vi "Not Equivalent.vi"(8 "Other JSON":string="{}", 10 "JSON":string="{}") -> (2 "Not Equivalent":bool caption="Not Equivalent (or invalid)")   [LabVIEW 2019, in "JSONtext.lvlib"]
doc: "Returns True if two JSON Values are \"Not Equivalent\".\n\nEqual means they are the same JSON infomation. Not considered differences are:\n -- different order of JSON Object items\n -- presence of any formating whitespace (outside of a JSON String)\n -- different formating of numbers (123.00 verus 123 or 1.23E2)\n\nNote: If using the LabVIEW extension that uses NaN numbers, these are considered Equivalent, ignoring the ususal convention of NaN not equal to NaN.\n\nInvalid JSON will always return \"Not Equivalent\" even if both inputs are identical.\n\nThis function looks only at the leading JSON Value in the input strings, ignoring any following characters."
uses:
  JSONtext.lvlib
  support/Get Number Text.vi
  String Subset.vi
  Parsing/Advance past Number.vi
  Parsing/Parsing Error in converting to LabVIEW type.vi
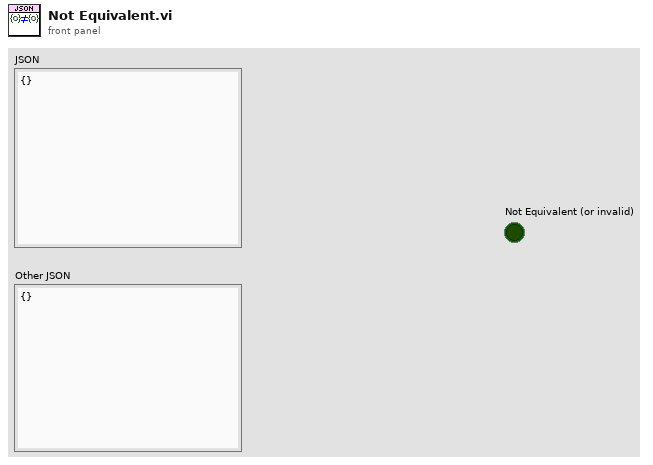
[diagram p1: front panel]
types:
  T1 = typedef "JSONtext.lvlib/JSON Value Type.ctl" = enum16{"Not a JSON Value", "JSON Object", "JSON Array", "String", "Number", "true", "false", "null"}
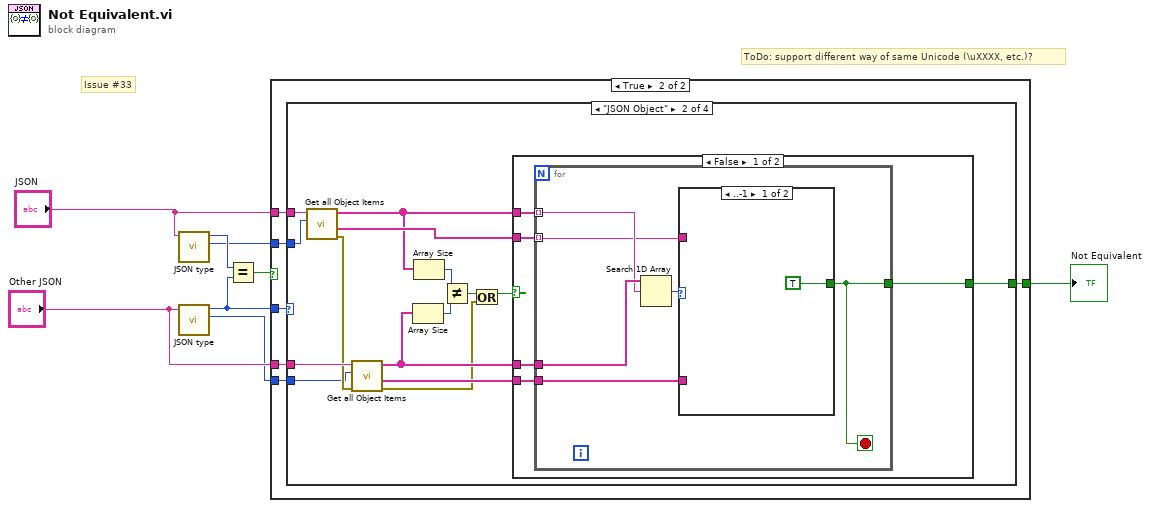
[diagram p0: block diagram]
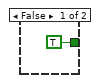
[diagram p2: hidden frame]
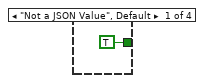
[diagram p3: hidden frame]
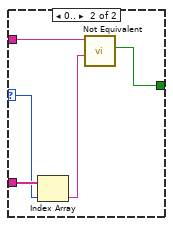
[diagram p4: hidden frame]
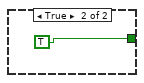
[diagram p5: hidden frame]
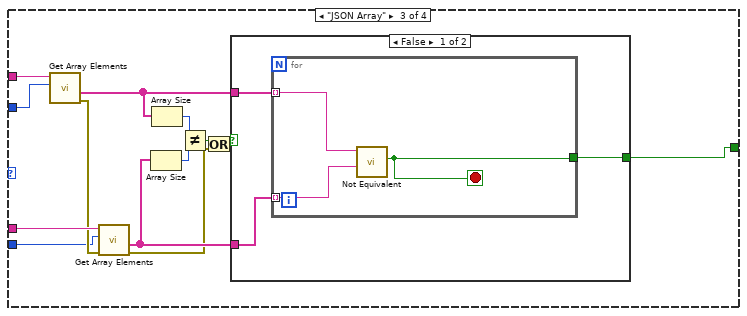
[diagram p6: hidden frame]
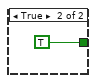
[diagram p7: hidden frame]
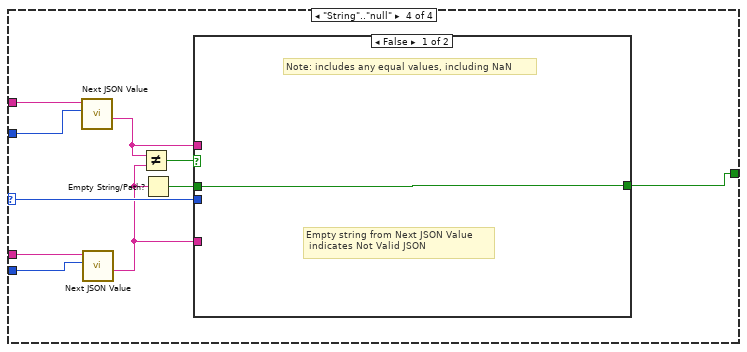
[diagram p8: hidden frame]
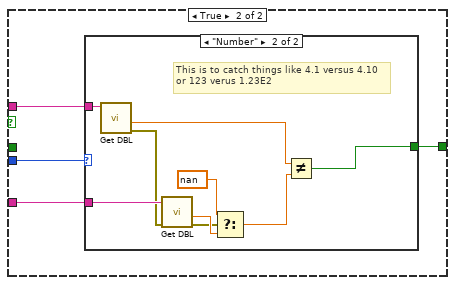
[diagram p9: hidden frame]
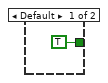
[diagram p10: hidden frame]
diagram:
  # "ToDo: support different way of same Unicode (\\uXXXX, etc.)?"
  # "Issue #33"
  n1 = call "JSON type.vi"("JSON"="JSON") -> ("Item Offset"=w1:i32, "JSON Value Type"=w5:T1)  [unwired: 9 in]
  n2 = call "JSON type.vi"("JSON"="Other JSON") -> ("Item Offset"=w2:i32, "JSON Value Type"=w3:T1)  [unwired: 9 in]
  n3 = Equal?(x=w5, y=w3) -> (x = y?=w4:bool)
  n4 = case shown="True" w4 {
    tunnel: "JSON" -> [_ w15]
    tunnel: "Other JSON" -> [_ w14]
    tunnel: w3 -> [_ w13]
    tunnel: [TRUE ("Not Equal") w12] -> w6
    tunnel: w2 -> [_ w11]
    tunnel: w1 -> [_ w10]
    frame False {
    }
    frame True {
      n5 = case shown="\"JSON Object\"" w13 {
        selector: w13 -> [_ _ _ w74]
        tunnel: w15 -> [_ w30 w62 w79]
        tunnel: w14 -> [_ w29 w61 w78]
        tunnel: [TRUE ("Not Equal") w21 w59 w77] -> w12
        tunnel: w11 -> [_ w17 w51 w75]
        tunnel: w10 -> [_ w18 w50 w76]
        frame "Not a JSON Value", Default {
        }
        frame "JSON Object" {
          n6 = call "Get all Object Items.vi"("Offset"=w18, "JSON"=w30) -> ("error out"=w27:errorcluster, "<JSON>"=w31:string[], "Item Names"=w26:string[])  [unwired: 6 in, 1 out]
          n7 = call "Get all Object Items.vi"("error in (no error)"=w27, "Offset"=w17, "JSON"=w29) -> ("error out"=w19:errorcluster, "<JSON>"=w28:string[], "Item Names"=w25:string[])  [unwired: 5 in, 1 out]
          n8 = Array Size(array=w25) -> (size(s)=w23:i32)
          n9 = Array Size(array=w26) -> (size(s)=w24:i32)
          n10 = Not Equal?(x=w24, y=w23) -> (x != y?=w22:bool)
          n11 = Or(x=w22, y=w19) -> (x .or. y?=w20:bool)
          n12 = case shown="False" w20 {
            tunnel: w31 -> [w36 _]
            tunnel: w28 -> [w35 _]
            tunnel: w26 -> [w34 _]
            tunnel: w25 -> [w33 _]
            tunnel: [w32 TRUE] -> w21
            frame False {
              n13 = for {
                tunnel: w34 -> [w39] mode=indexing
                tunnel: w33 -> [w42]
                tunnel: w36 -> [w38] mode=indexing
                tunnel: w35 -> [w40]
                tunnel: [w37] -> w32
                stop <- w37 stop-if-true
                n14 = Search 1D Array(1D array=w42, element=w39) -> (index of element=w41:i32)  [unwired: 1 in]
                n15 = case shown="..-1" w41 {
                  selector: w41 -> [_ w47]
                  tunnel: w38 -> [_ w45]
                  tunnel: w40 -> [_ w48]
                  tunnel: [TRUE ("Not Equivalent") w44] -> w37
                  frame ..-1 {
                  }
                  frame 0.. {
                    n16 = Index Array(array=w48, index=w47) -> (element=w46:string)
                    n17 = call "Not Equivalent.vi"("Other JSON"=w46, "JSON"=w45) -> ("Not Equivalent"=w44:bool)  [unwired: 8 in]
                  }
                }
              }
            }
            frame True {
            }
          }
        }
        frame "JSON Array" {
          n18 = call "Get Array Elements.vi"("Offset"=w50, "JSON"=w62) -> ("error out"=w60:errorcluster, "<JSON>"=w56:string[])  [unwired: 7 in, 1 out]
          n19 = call "Get Array Elements.vi"("error in (no error)"=w60, "Offset"=w51, "JSON"=w61) -> ("error out"=w52:errorcluster, "<JSON>"=w55:string[])  [unwired: 6 in, 1 out]
          n20 = Array Size(array=w55) -> (size(s)=w57:i32)
          n21 = Array Size(array=w56) -> (size(s)=w58:i32)
          n22 = Not Equal?(x=w58, y=w57) -> (x != y?=w54:bool)
          n23 = Or(x=w54, y=w52) -> (x .or. y?=w53:bool)
          n24 = case shown="False" w53 {
            tunnel: [w63 TRUE] -> w59
            tunnel: w56 -> [w65 _]
            tunnel: w55 -> [w64 _]
            frame False {
              n25 = for {
                tunnel: w65 -> [w68] mode=indexing
                tunnel: w64 -> [w67] mode=indexing
                tunnel: [w66] -> w63
                stop <- w66 stop-if-true
                n26 = call "Not Equivalent.vi"("Other JSON"=w67, "JSON"=w68) -> ("Not Equivalent"=w66:bool)  [unwired: 8 in]
              }
            }
            frame True {
            }
          }
        }
        frame "String".."null" {
          n27 = call "Next JSON Value.vi"("Offset"=w76, "JSON"=w79) -> ("<JSON>"=w73:string)  [unwired: 6 in, 3 out]
          n28 = call "Next JSON Value.vi"("Offset"=w75, "JSON"=w78) -> ("<JSON>"=w71:string)  [unwired: 6 in, 3 out]
          n29 = Not Equal?(x=w73, y=w71) -> (x != y?=w72:bool)
          n30 = Empty String/Path?(string/path=w71) -> (empty?=w70:bool)
          n31 = case shown="False" w72 {
            tunnel: [w80 w82] -> w77
            tunnel: w73 -> [_ w84]
            tunnel: w71 -> [_ w83]
            tunnel: w74 -> [_ w81]
            tunnel: w70 -> [w80 _]
            frame False {
              # "Empty string from Next JSON Value\n indicates Not Valid JSON"
              # "Note: includes any equal values, including NaN"
            }
            frame True {
              n32 = case shown="\"Number\"" w81 {
                tunnel: w84 -> [_ w94]
                tunnel: w83 -> [_ w90]
                tunnel: [TRUE w86] -> w82
                frame Default {
                }
                frame "Number" {
                  # "This is to catch things like 4.1 versus 4.10\nor 123 verus 1.23E2"
                  n33 = call "Get DBL.vi"("JSON"=w94) -> ("error out"=w89:errorcluster, "Number"=w87:dbl)  [unwired: 8 in, 1 out]
                  n34 = call "Get DBL.vi"("error in (no error)"=w89, "JSON"=w90) -> ("error out"=w91:errorcluster, "Number"=w92:dbl)  [unwired: 7 in, 1 out]
                  n35 = Select(t=nan, s=w91, f=w92) -> (s? t:f=w88:dbl)
                  n36 = Not Equal?(x=w87, y=w88) -> (x != y?=w86:bool)
                }
              }
            }
          }
        }
      }
    }
  }
  "Not Equivalent" <- w6
